vi "Decode Status Byte.vi"(0 "Status Byte":T1) -> (1 "Mode":enum8{"Tele-Op", "Auto", ""}(ring)=enum."", 2 "Status":T2(ring))   [LabVIEW 2012]
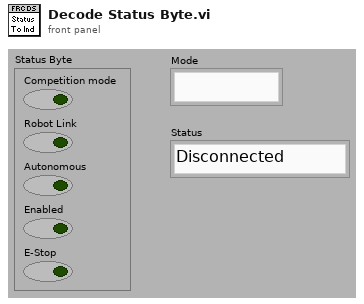
[diagram p1: front panel]
types:
  T1 = cluster{"Competition mode":bool, "Robot Link":bool, "Autonomous":bool, "Enabled":bool, "E-Stop":bool}
  T2 = enum8{"Disconnected", "E-Stop", "Disabled", "Enabled"}
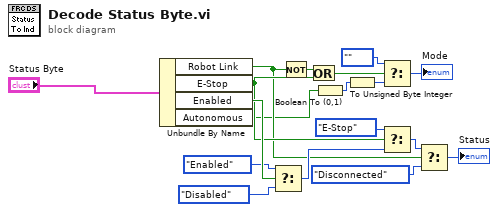
[diagram p0: block diagram]
diagram:
  n1 = Unbundle By Name("Status Byte") -> ("Robot Link"=w9:bool, "E-Stop"=w14:bool, "Enabled"=w18:bool, "Autonomous"=w3:bool)
  n2 = Select(t=T2."Enabled" ("Status"), s=w18, f=T2."Disabled" ("Status")) -> (s? t:f=w15:T2)
  n3 = Not(x=w9) -> (.not. x?=w2:bool)
  n4 = Or(x=w2, y=w14) -> (x .or. y?=w4:bool)
  n5 = Boolean To (0,1)(Boolean=w3) -> (0, 1=w6:i16)
  n6 = To Unsigned Byte Integer(number=w6) -> (unsigned 8bit integer=w8:u8)
  n7 = Select(t=enum8{"Tele-Op", "Auto", ""}."" ("Mode"), s=w4, f=w8) -> (s? t:f=→"Mode":u8)
  n8 = Select(t=T2."E-Stop" ("Status"), s=w14, f=w15) -> (s? t:f=w12:T2)
  n9 = Select(t=w12, s=w9, f=T2."Disconnected" ("Status")) -> (s? t:f=→"Status":T2)
